vi "n to sn.vi"(1 "in":string) -> (0 "out":string)   [LabVIEW 2017, in "Error File Management.lvlib"]
uses:
  Error File Management.lvlib
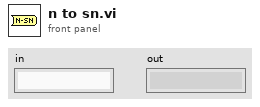
[diagram p1: front panel]
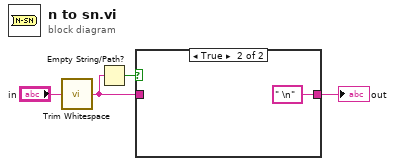
[diagram p0: block diagram]
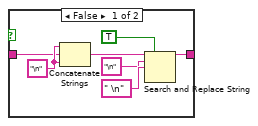
[diagram p2: hidden frame]
diagram:
  n1 = call <vilib>:"Trim Whitespace.vi"("string"="in") -> ("trimmed string"=w3:string)  [unwired: 1 in]
  n2 = Empty String/Path?(string/path=w3) -> (empty?=w4:bool)
  n3 = case shown="True" w4 {
    tunnel: [w10 " \n" ("search string")] -> w1
    tunnel: w3 -> [w5 _]
    frame False {
      w6 = "\n" ("search string")
      n4 = Concatenate Strings(w6, w5, w6) -> (w7:string)
      n5 = Search and Replace String(replace all?=TRUE ("replace all? (F)"), input string=w7, search string="\n", replace string=" \n" ("search string")) -> (result string=w10:string)  [unwired: 4 in, 3 out]
    }
    frame True {
    }
  }
  "out" <- w1
